vi "Report Pump State.vi"(8 "error in (no error)":cluster{"状态":bool, "代码":i32, "源":string} caption="错误输入（无错误）", 10 "泵状态":bool, 11 "蒸发冷却器输入":refnum<class "Evaporative Cooler.lvclass">) -> (0 "error out":cluster{"状态":bool, "代码":i32, "源":string} caption="错误输出")   [LabVIEW 2013, in "Evaporative Cooler.lvlib" / "Evaporative Cooler.lvclass"]
doc: "向控制器发送消息，通知泵的状态（打开或关闭）。"
uses:
  Evaporative Cooler.lvclass
  <vilib>/ActorFramework/Message Enqueuer/Message Enqueuer.lvclass
  Cooler/Cooler/Cooler.lvclass/Cooler.ctl
  Evaporative Cooler Controller/Update Pump State Msg/Update Pump State Msg.lvclass/Update Pump State Msg.ctl
  <vilib>/ActorFramework/Message Enqueuer/Message Enqueuer.lvclass/Message Enqueuer.ctl
  <vilib>/ActorFramework/Message Enqueuer/Enqueue.vi
  <vilib>/ActorFramework/Message Priority Queue/Priority Enqueue.vi
  Evaporative Cooler Controller/Update Pump State Msg/Update Pump State Msg.lvclass
  Cooler/Cooler/Cooler.lvclass
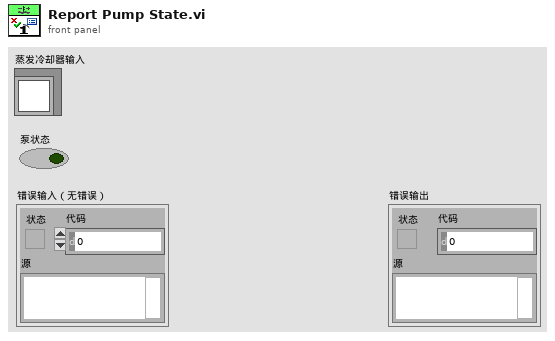
[diagram p1: front panel]
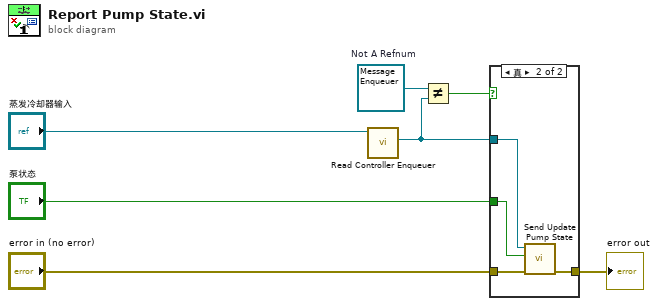
[diagram p0: block diagram]
diagram:
  w2 = refnum<class "Message Enqueuer.lvclass"> refnum  # Not A Refnum
  n1 = call "Read Controller Enqueuer.vi"("冷却器"="蒸发冷却器输入") -> ("控制器待入队列"=w3:refnum<class "Message Enqueuer.lvclass">)  [unwired: 10 in]
  n2 = Not Equal?(x=w2, y=w3) -> (x != y?=w1:bool)
  n3 = case shown="真" w1 {
    tunnel: "泵状态" -> [_ w12]
    tunnel: [w8 w11] -> w5
    tunnel: w3 -> [_ w10]
    tunnel: "error in (no error)" -> [w8 w9]
    frame False {
    }
    frame True {
      n4 = call "Send Update Pump State.vi"("error in (no error)"=w9, "泵打开？"=w12, "消息待入队列"=w10) -> ("error out"=w11:cluster{"状态":bool, "代码":i32, "源":string})  [unwired: 8 in]
    }
  }
  "error out" <- w5
